vi "Read Run.vi"(11 "DAQ in":refnum<class "DAQ.lvclass">) -> (2 "Run":refnum<user-event>, 3 "DAQ out":refnum<class "DAQ.lvclass">)   [LabVIEW 2011, in "DAQ.lvclass"]
uses:
  DAQ.lvclass
  DAQ.lvclass/DAQ.ctl
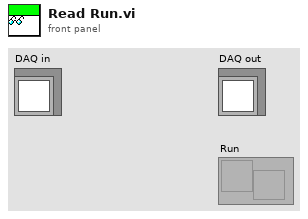
[diagram p1: front panel]
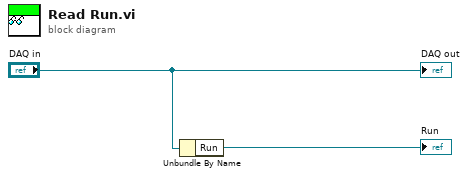
[diagram p0: block diagram]
diagram:
  n1 = Unbundle By Name("DAQ in") -> ("Run"=→"Run":refnum<user-event>)
  "DAQ out" <- "DAQ in"
